vi "act 20.vi"   [LabVIEW 2010]
uses:
  act/lv_07/lv_07.lvlib
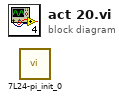
[diagram p0: block diagram]
diagram:
  n1 = call "7L24-pi_init_0.vi"() -> ()  [unwired: 2 in, 2 out]
